vi "SeparateLinesHTML.vi"(9 "Line end marker":string, 10 "Line start marker":string, 11 "Input String":string) -> (1 "End of Sting ?":bool, 2 "Line Out":string, 3 "Remaining String":string)   [LabVIEW 2017, in "DS_Lib.lvlib" / "SRNotesParser.lvlib"]
uses:
  SRNotesParser.lvlib
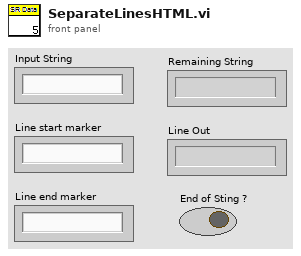
[diagram p1: front panel]
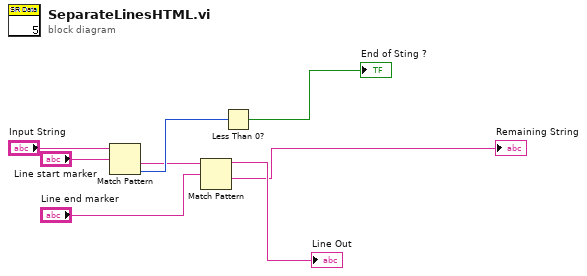
[diagram p0: block diagram]
diagram:
  n1 = Match Pattern(string="Input String", regular expression="Line start marker") -> (after substring=w3:string, offset past match=w5:i32)  [unwired: 1 in, 2 out]
  n2 = Match Pattern(string=w3, regular expression="Line end marker") -> (before substring=→"Line Out":string, after substring=→"Remaining String":string)  [unwired: 1 in, 2 out]
  n3 = Less Than 0?(x=w5) -> (x < 0?=→"End of Sting ?":bool)
